vi "Клиент MotorSPS.vi"() -> ()   [LabVIEW 2010]
uses:
  <vilib>/Utility/miscctls.llb/LVScalePositionTypeDef.ctl
  <vilib>/Utility/miscctls.llb/LVRemotePanelConnectionsTypeDef.ctl
panel:
  out "Remote Panel Connections":T1
  out "Remote Panel Controller":i32
  out "VariableIn":T3
  in  "machine name (\"\":  open local reference)":string
  in  "MotorSPS":T4={"Ручной режим управления"={"РучнойСтартСтоп"=FALSE, "Напраление вращения"=enum."Лево", "Время в мин"=18.0, "Поворт экрана"=180.0, "СкорРучРежМот"=0.0, "СкорРучРежРед"=0.0, "Значение энкодера"=0.0, "Расчитать скорость"=FALSE, "Способ управления СПШ"=enum."Управления позицией", "Контроль энкодера"=FALSE, "Инкремент импульсов"=0.0, "Условие энкодер"=FALSE, "Контроль времени"=FALSE, "Лимит времени"=0.0, "Условие время"=FALSE, "Контроль концевиков"=TRUE, "Начальная позиция"=0.0, "Текущая позиция"=0.0, "Выбег"=0.0, "Заданная позиция"=0.0, "Пуск Руч"=FALSE, "Стоп Руч"=FALSE}, "Поиск нулевого положения"={"ИсхСостСтарСтоп"=FALSE, "КонтрольКон"=enum."КонтрольПравКон", "SpeeSlide"=0.0, "Скорость двигателя"=0.0, "Скорость редуктора"=0.0, "Двигатель в исходное сотояние"=FALSE}, "Прав.Конц"=FALSE, "Лев.Конц"=FALSE, "GaugeAngle"={0.0, 0.0}, "Индикатор Статуса Конт"=FALSE, "Статус контроллера СПШ"=enum."Исправен", "Журнал событий"=0, "Выход из программы"=FALSE, "timestamp"=timestamp(0 s since 1904-01-01)} {"timestamp" format="%<%H:%M:%S%3u     %d.%m.%Y>T"; "Поиск нулевого положения"."Скорость двигателя" min=0.0 max=200.0 step=5.0; "Поиск нулевого положения"."SpeeSlide" step=5.0 scale=0.0..200.0; "Ручной режим управления"."Лимит времени" format="%<%M:%S>T"; "Ручной режим управления"."СкорРучРежРед" format="%#_g об/мин"; "Ручной режим управления"."Поворт экрана" min=0.0 max=360.0 step=1.0 format="%#_g °"; "Ручной режим управления"."Время в мин" min=1.0 max=60.0 step=1.0 format="%2d мин"; "Ручной режим управления"."СкорРучРежМот" format="%#_g об/мин"}
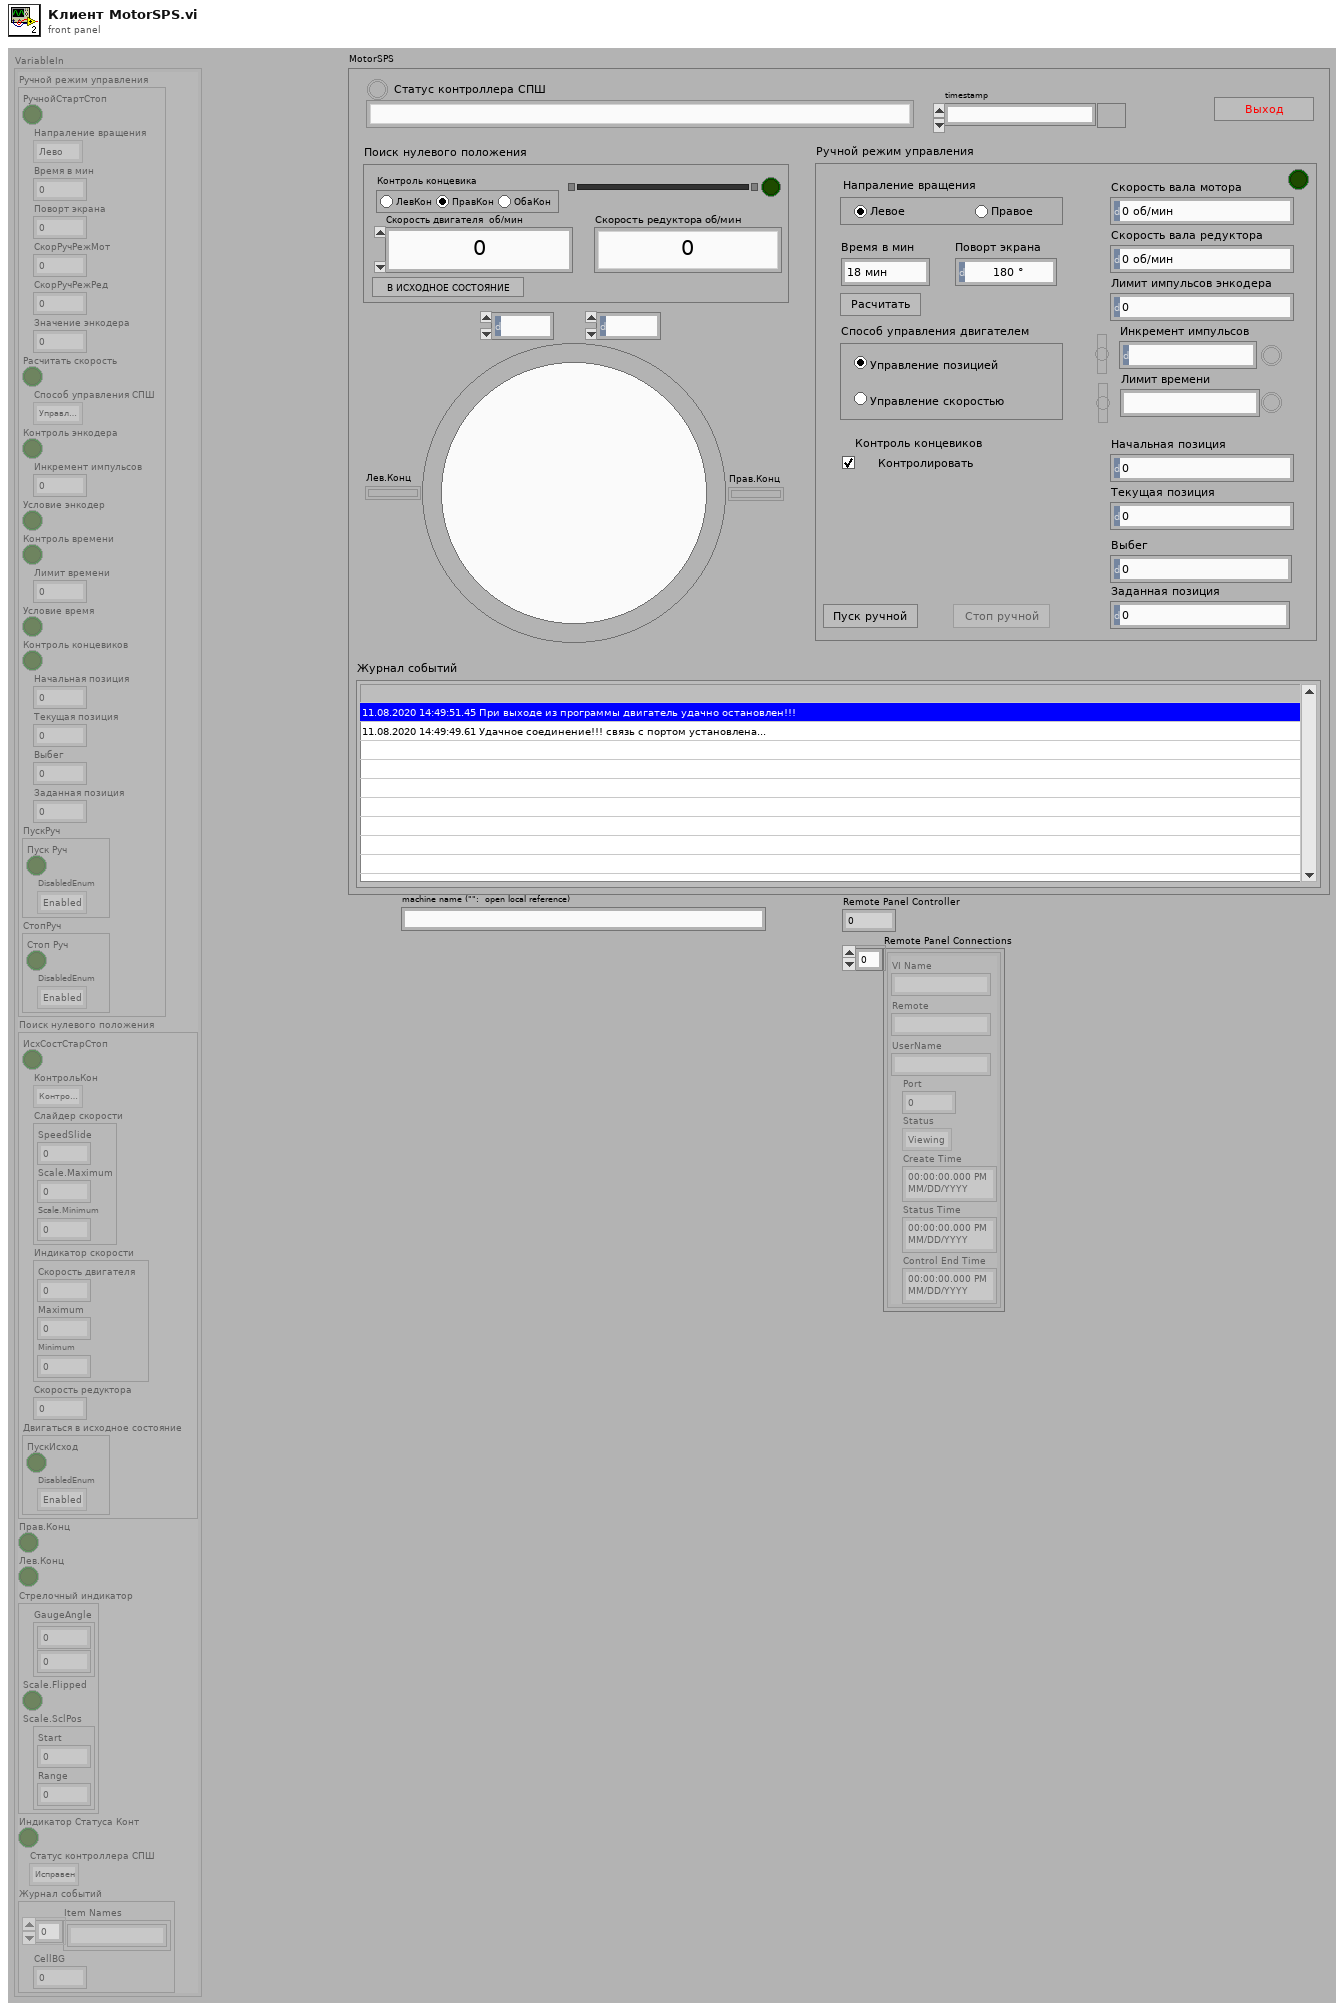
[diagram p1: front panel]
types:
  T1 = typedef "LVRemotePanelConnectionsTypeDef.ctl" = cluster{"VI Name":string, "Remote":string, "UserName":string, "Port":i32, "Status":enum32{"Viewing", "Waiting For Control", "Controlling"}, "Create Time":timestamp, "Status Time":timestamp, "Control End Time":timestamp}[]
  T2 = typedef "LVScalePositionTypeDef.ctl" = cluster{"Start":dbl, "Range":dbl}
  T3 = cluster{"Ручной режим управления":cluster{"РучнойСтартСтоп":bool, "Напраление вращения":enum32{"Лево", "Право"}, "Время в мин":dbl, "Поворт экрана":dbl, "СкорРучРежМот":dbl, "СкорРучРежРед":dbl, "Значение энкодера":dbl, "Расчитать скорость":bool, "Способ управления СПШ":enum32{"Управления позицией", "Управления скоростью"}, "Контроль энкодера":bool, "Инкремент импульсов":dbl, "Условие энкодер":bool, "Контроль времени":bool, "Лимит времени":dbl, "Условие время":bool, "Контроль концевиков":bool, "Начальная позиция":dbl, "Текущая позиция":dbl, "Выбег":dbl, "Заданная позиция":dbl, "ПускРуч":cluster{"Пуск Руч":bool, "DisabledEnum":enum8{"Enabled", "Disabled", "Disabled and Grayed Out"}}, "СтопРуч":cluster{"Стоп Руч":bool, "DisabledEnum":enum8{"Enabled", "Disabled", "Disabled and Grayed Out"}}}, "Поиск нулевого положения":cluster{"ИсхСостСтарСтоп":bool, "КонтрольКон":enum32{"КонтрольЛевКон", "КонтрольПравКон", "КонтрольОбаКон"}, "Слайдер скорости":cluster{"SpeedSlide":dbl, "Scale.Maximum":dbl, "Scale.Minimum":dbl}, "Индикатор скорости":cluster{"Скорость двигателя":dbl, "Maximum":dbl, "Minimum":dbl}, "Скорость редуктора":dbl, "Двигаться в исходное состояние":cluster{"ПускИсход":bool, "DisabledEnum":enum8{"Enabled", "Disabled", "Disabled and Grayed Out"}}}, "Прав.Конц":bool, "Лев.Конц":bool, "Стрелочный индикатор":cluster{"GaugeAngle":cluster{dbl, dbl}, "Scale.Flipped":bool, "Scale.SclPos":T2}, "Индикатор Статуса Конт":bool, "Статус контроллера СПШ":enum16{"Исправен", "Останов по команде", "Останов - высокое противодействующее усилие", "Останов - короткое замыкангие", "Выход из температурного диапазона", "Повышенное силовое напряжение", "Низкое силовое напряжение", "Повышанное цифровое напряжение", "Низкое цифровое напряжение", "Силовое напряжение превышает напряжение, установленое пользователем", "Останов - превышение допустимой перегрузки", "Останов - сработала защита IGBT модуля", "Останов - ощибка поиска фаз по UVW трекам", "Останов - ошибка в настройках энкодера", "Останов - сбой в работе энкодера", "Останов - ошибка фазировки двигателя"}, "Журнал событий":cluster{"Item Names":string[], "CellBG":u32}}
  T4 = cluster{"Ручной режим управления":cluster{"РучнойСтартСтоп":bool, "Напраление вращения":enum32{"Лево", "Право"}, "Время в мин":dbl, "Поворт экрана":dbl, "СкорРучРежМот":dbl, "СкорРучРежРед":dbl, "Значение энкодера":dbl, "Расчитать скорость":bool, "Способ управления СПШ":enum32{"Управления позицией", "Управления скоростью"}, "Контроль энкодера":bool, "Инкремент импульсов":dbl, "Условие энкодер":bool, "Контроль времени":bool, "Лимит времени":dbl, "Условие время":bool, "Контроль концевиков":bool, "Начальная позиция":dbl, "Текущая позиция":dbl, "Выбег":dbl, "Заданная позиция":dbl, "Пуск Руч":bool, "Стоп Руч":bool}, "Поиск нулевого положения":cluster{"ИсхСостСтарСтоп":bool, "КонтрольКон":enum32{"КонтрольЛевКон", "КонтрольПравКон", "КонтрольОбаКон"}, "SpeeSlide":dbl, "Скорость двигателя":dbl, "Скорость редуктора":dbl, "Двигатель в исходное сотояние":bool}, "Прав.Конц":bool, "Лев.Конц":bool, "GaugeAngle":cluster{dbl, dbl}, "Индикатор Статуса Конт":bool, "Статус контроллера СПШ":enum16{"Исправен", "Останов по команде", "Останов - высокое противодействующее усилие", "Останов - короткое замыкангие", "Выход из температурного диапазона", "Повышенное силовое напряжение", "Низкое силовое напряжение", "Повышанное цифровое напряжение", "Низкое цифровое напряжение", "Силовое напряжение превышает напряжение, установленое пользователем", "Останов - превышение допустимой перегрузки", "Останов - сработала защита IGBT модуля", "Останов - ощибка поиска фаз по UVW трекам", "Останов - ошибка в настройках энкодера", "Останов - сбой в работе энкодера", "Останов - ошибка фазировки двигателя"}, "Журнал событий":i32, "Выход из программы":bool, "timestamp":timestamp}
  T5 = cluster{"ИсхСостСтарСтоп":bool, "КонтрольКон":enum32{"КонтрольЛевКон", "КонтрольПравКон", "КонтрольОбаКон"}, "Слайдер скорости":cluster{"SpeedSlide":dbl, "Scale.Maximum":dbl, "Scale.Minimum":dbl}, "Индикатор скорости":cluster{"Скорость двигателя":dbl, "Maximum":dbl, "Minimum":dbl}, "Скорость редуктора":dbl, "Двигаться в исходное состояние":cluster{"ПускИсход":bool, "DisabledEnum":enum8{"Enabled", "Disabled", "Disabled and Grayed Out"}}}
  T6 = cluster{"GaugeAngle":cluster{dbl, dbl}, "Scale.Flipped":bool, "Scale.SclPos":T2}
  T7 = cluster{"РучнойСтартСтоп":bool, "Напраление вращения":enum32{"Лево", "Право"}, "Время в мин":dbl, "Поворт экрана":dbl, "СкорРучРежМот":dbl, "СкорРучРежРед":dbl, "Значение энкодера":dbl, "Расчитать скорость":bool, "Способ управления СПШ":enum32{"Управления позицией", "Управления скоростью"}, "Контроль энкодера":bool, "Инкремент импульсов":dbl, "Условие энкодер":bool, "Контроль времени":bool, "Лимит времени":dbl, "Условие время":bool, "Контроль концевиков":bool, "Начальная позиция":dbl, "Текущая позиция":dbl, "Выбег":dbl, "Заданная позиция":dbl, "ПускРуч":cluster{"Пуск Руч":bool, "DisabledEnum":enum8{"Enabled", "Disabled", "Disabled and Grayed Out"}}, "СтопРуч":cluster{"Стоп Руч":bool, "DisabledEnum":enum8{"Enabled", "Disabled", "Disabled and Grayed Out"}}}
  T8 = enum16{"Исправен", "Останов по команде", "Останов - высокое противодействующее усилие", "Останов - короткое замыкангие", "Выход из температурного диапазона", "Повышенное силовое напряжение", "Низкое силовое напряжение", "Повышанное цифровое напряжение", "Низкое цифровое напряжение", "Силовое напряжение превышает напряжение, установленое пользователем", "Останов - превышение допустимой перегрузки", "Останов - сработала защита IGBT модуля", "Останов - ощибка поиска фаз по UVW трекам", "Останов - ошибка в настройках энкодера", "Останов - сбой в работе энкодера", "Останов - ошибка фазировки двигателя"}
  T9 = enum32{"КонтрольЛевКон", "КонтрольПравКон", "КонтрольОбаКон"}
  T10 = enum8{"Enabled", "Disabled", "Disabled and Grayed Out"}
  T11 = enum32{"Управления позицией", "Управления скоростью"}
  T12 = cluster{"ИсхСостСтарСтоп":bool, "КонтрольКон":enum32{"КонтрольЛевКон", "КонтрольПравКон", "КонтрольОбаКон"}, "SpeeSlide":dbl, "Скорость двигателя":dbl, "Скорость редуктора":dbl, "Двигатель в исходное сотояние":bool}
  T13 = cluster{"РучнойСтартСтоп":bool, "Напраление вращения":enum32{"Лево", "Право"}, "Время в мин":dbl, "Поворт экрана":dbl, "СкорРучРежМот":dbl, "СкорРучРежРед":dbl, "Значение энкодера":dbl, "Расчитать скорость":bool, "Способ управления СПШ":enum32{"Управления позицией", "Управления скоростью"}, "Контроль энкодера":bool, "Инкремент импульсов":dbl, "Условие энкодер":bool, "Контроль времени":bool, "Лимит времени":dbl, "Условие время":bool, "Контроль концевиков":bool, "Начальная позиция":dbl, "Текущая позиция":dbl, "Выбег":dbl, "Заданная позиция":dbl, "Пуск Руч":bool, "Стоп Руч":bool}
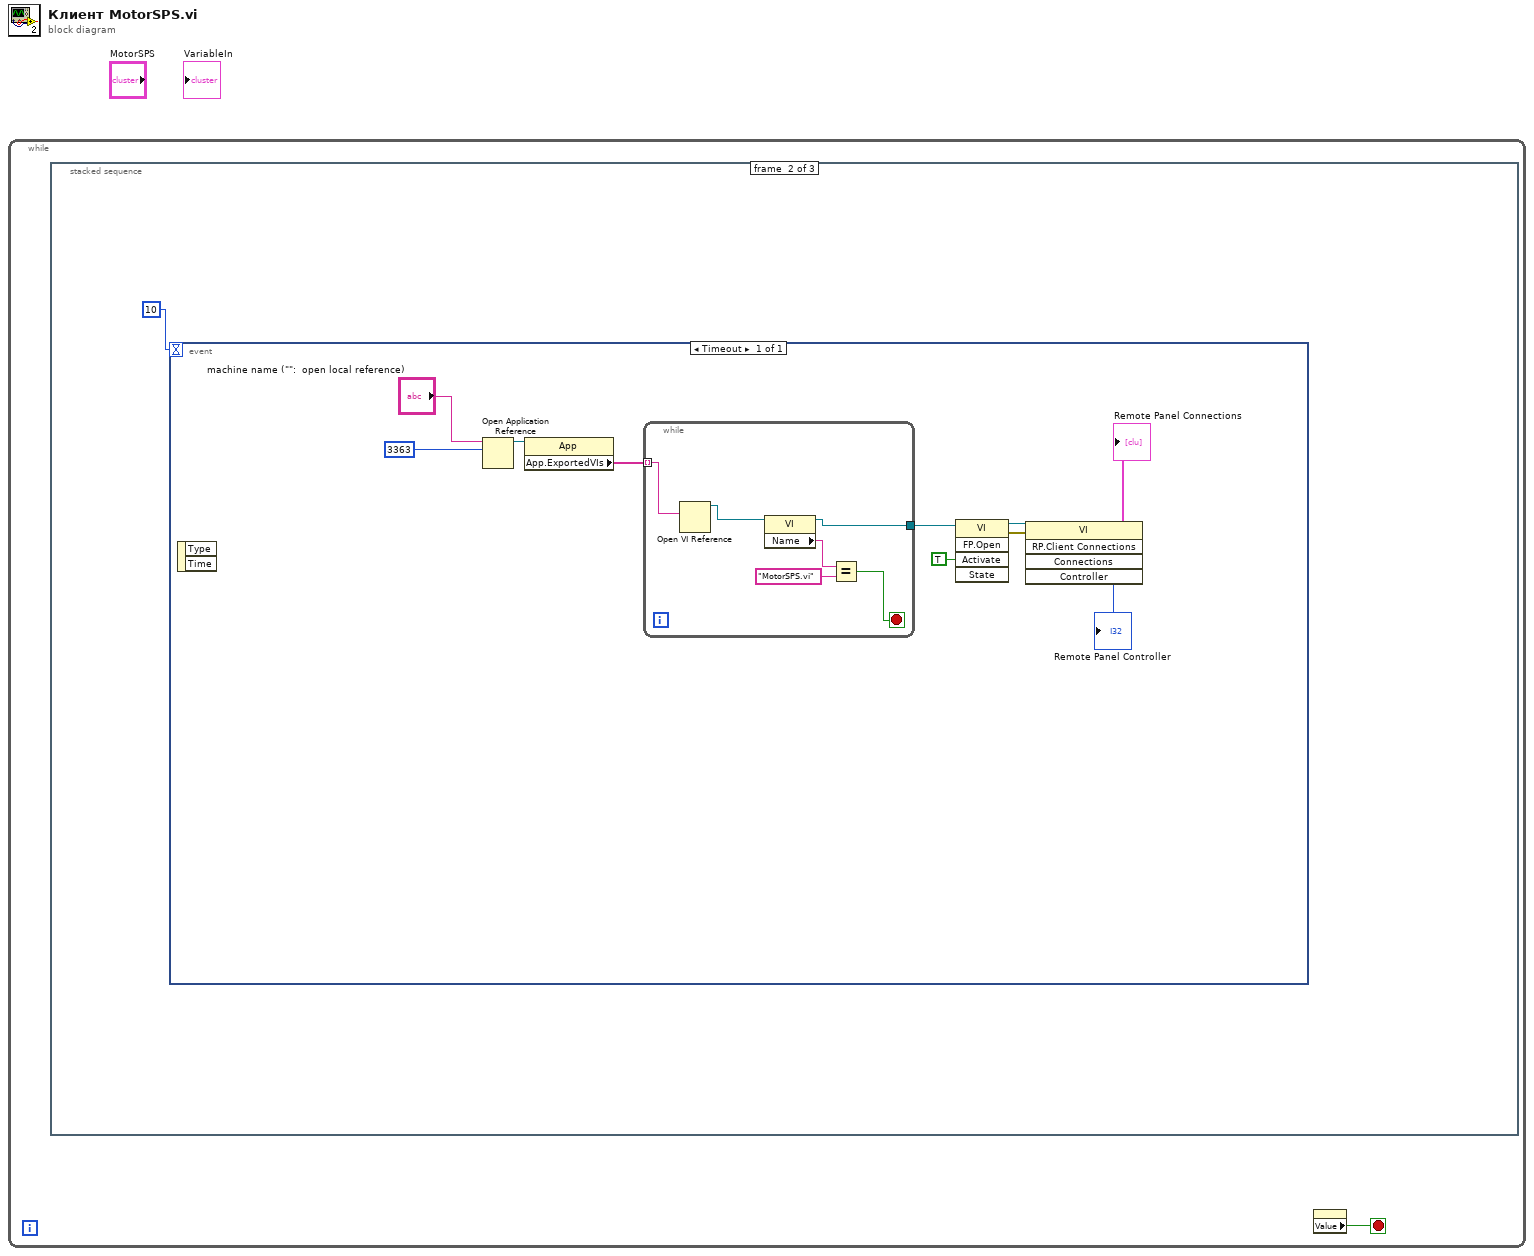
[diagram p0: block diagram]
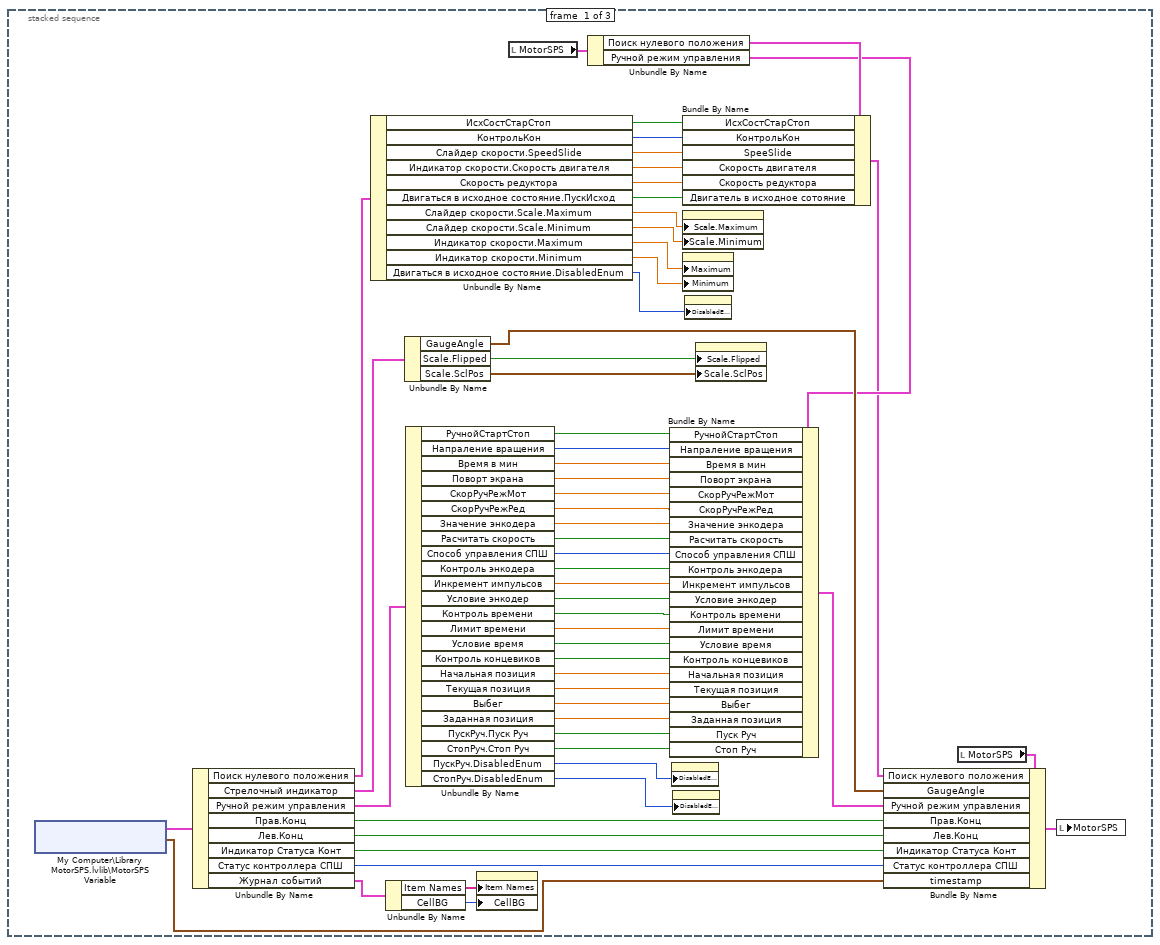
[diagram p2: hidden frame]
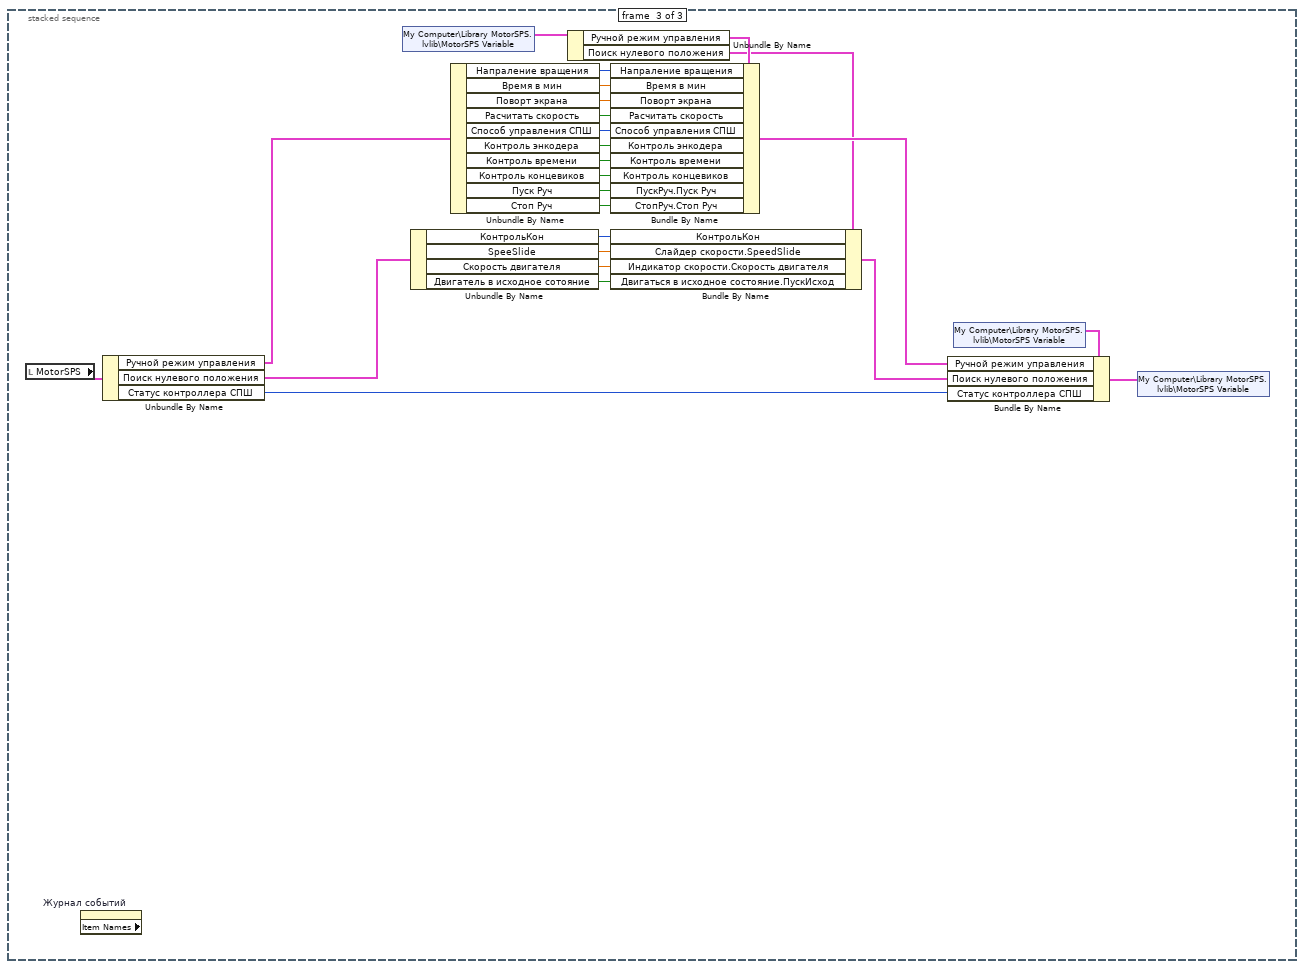
[diagram p3: hidden frame]
diagram:
  n1 = while {
    stop <- w1 stop-if-true
    n2 = stacked-sequence {
      frame #0 {
        n3 = shared-variable "My Computer\\Library MotorSPS.lvlib\\MotorSPS Variable"() -> (w8:T3, w7:timestamp)  [unwired: 1 in, 1 out]
        n4 = Unbundle By Name(w8) -> ("Поиск нулевого положения"=w41:T5, "Стрелочный индикатор"=w40:T6, "Ручной режим управления"=w33:T7, "Прав.Конц"=w37:bool, "Лев.Конц"=w36:bool, "Индикатор Статуса Конт"=w56:bool, "Статус контроллера СПШ"=w55:T8, "Журнал событий"=w54:cluster{"Item Names":string[], "CellBG":u32})
        n5 = Unbundle By Name(w41) -> ("ИсхСостСтарСтоп"=w51:bool, "КонтрольКон"=w50:T9, "Слайдер скорости.SpeedSlide"=w49:dbl, "Индикатор скорости.Скорость двигателя"=w48:dbl, "Скорость редуктора"=w47:dbl, "Двигаться в исходное состояние.ПускИсход"=w46:bool, "Слайдер скорости.Scale.Maximum"=w45:dbl, "Слайдер скорости.Scale.Minimum"=w44:dbl, "Индикатор скорости.Maximum"=w43:dbl, "Индикатор скорости.Minimum"=w42:dbl, "Двигаться в исходное состояние.DisabledEnum"=w35:T10)
        n6 = Unbundle By Name(w54) -> ("Item Names"=w53:string[], "CellBG"=w52:u32)
        n7 = Unbundle By Name(w40) -> ("GaugeAngle"=w39:cluster{dbl, dbl}, "Scale.Flipped"=w38:bool, "Scale.SclPos"=w34:T2)
        n8 = Unbundle By Name(w33) -> ("РучнойСтартСтоп"=w32:bool, "Напраление вращения"=w31:enum32{"Лево", "Право"}, "Время в мин"=w30:dbl, "Поворт экрана"=w29:dbl, "СкорРучРежМот"=w28:dbl, "СкорРучРежРед"=w27:dbl, "Значение энкодера"=w26:dbl, "Расчитать скорость"=w25:bool, "Способ управления СПШ"=w24:T11, "Контроль энкодера"=w23:bool, "Инкремент импульсов"=w22:dbl, "Условие энкодер"=w21:bool, "Контроль времени"=w20:bool, "Лимит времени"=w19:dbl, "Условие время"=w18:bool, "Контроль концевиков"=w17:bool, "Начальная позиция"=w16:dbl, "Текущая позиция"=w15:dbl, "Выбег"=w14:dbl, "Заданная позиция"=w13:dbl, "ПускРуч.Пуск Руч"=w12:bool, "СтопРуч.Стоп Руч"=w11:bool, "ПускРуч.DisabledEnum"=w10:T10, "СтопРуч.DisabledEnum"=w9:T10)
        n9 = property on="Журнал событий" class="LstBox (strict)"("Item Names"=w53, "CellBG"=w52) -> ()  [unwired: 2 in, 2 out]
        n10 = local read "MotorSPS"() -> (w6:T4)
        n11 = Unbundle By Name(w6) -> ("Поиск нулевого положения"=w5:T12, "Ручной режим управления"=w4:T13)
        n12 = Bundle By Name(cluster=w4, "РучнойСтартСтоп"=w32, "Напраление вращения"=w31, "Время в мин"=w30, "Поворт экрана"=w29, "СкорРучРежМот"=w28, "СкорРучРежРед"=w27, "Значение энкодера"=w26, "Расчитать скорость"=w25, "Способ управления СПШ"=w24, "Контроль энкодера"=w23, "Инкремент импульсов"=w22, "Условие энкодер"=w21, "Контроль времени"=w20, "Лимит времени"=w19, "Условие время"=w18, "Контроль концевиков"=w17, "Начальная позиция"=w16, "Текущая позиция"=w15, "Выбег"=w14, "Заданная позиция"=w13, "Пуск Руч"=w12, "Стоп Руч"=w11) -> (w3:T13)
        n13 = property on="Пуск Руч" class="Bool (strict)"("DisabledEnum"=w10) -> ()  [unwired: 2 in, 2 out]
        n14 = property on="Стоп Руч" class="Bool (strict)"("DisabledEnum"=w9) -> ()  [unwired: 2 in, 2 out]
        n15 = Bundle By Name(cluster=w5, "ИсхСостСтарСтоп"=w51, "КонтрольКон"=w50, "SpeeSlide"=w49, "Скорость двигателя"=w48, "Скорость редуктора"=w47, "Двигатель в исходное сотояние"=w46) -> (w2:T12)
        n16 = property on="SpeeSlide" class="Slide (strict)"("Scale.Maximum"=w45, "Scale.Minimum"=w44) -> ()  [unwired: 2 in, 2 out]
        n17 = property on="Скорость двигателя" class="DigNum (strict)"("Maximum"=w43, "Minimum"=w42) -> ()  [unwired: 2 in, 2 out]
        n18 = property on="Двигатель в исходное сотояние" class="Bool (strict)"("DisabledEnum"=w35) -> ()  [unwired: 2 in, 2 out]
        n19 = property on="GaugeAngle" class="Knob (strict)"("Scale.Flipped"=w38, "Scale.SclPos"=w34) -> ()  [unwired: 2 in, 2 out]
        n20 = local read "MotorSPS"() -> (w57:T4)
        n21 = Bundle By Name(cluster=w57, "Поиск нулевого положения"=w2, "GaugeAngle"=w39, "Ручной режим управления"=w3, "Прав.Конц"=w37, "Лев.Конц"=w36, "Индикатор Статуса Конт"=w56, "Статус контроллера СПШ"=w55, "timestamp"=w7) -> (w58:T4)
        n22 = local write "MotorSPS"(w58) -> ()
      }
      frame #1 {
        n23 = event shown="[0] Timeout" {
          selector: _ -> [_]
          dyn-events: _ -> [_]
          timeout: 10 -> [_]
          event Timeout {
            n24 = event-data() -> ()  [unwired: 1 in, 2 out]
            n25 = Open Application Reference(10:u16 3363 ("port number or service name (3363)"), 11:"machine name (\"\":  open local reference)") -> (3:w67:refnum<vi>)  [unwired: 2 in, 1 out]
            n26 = property class="App"(reference=w67) -> ("App.ExportedVIs"=w66:string[])  [unwired: 1 in, 2 out]
            n27 = while {
              tunnel: w66 -> [w75] mode=indexing
              tunnel: [w70] -> w65
              stop <- w71 stop-if-true
              n28 = Open VI Reference(vi path=w75) -> (vi reference=w74:refnum<vi>)  [unwired: 5 in, 1 out]
              n29 = property class="VI"(reference=w74) -> (reference out=w70:refnum<vi>, "Name"=w73:string)  [unwired: 1 in, 1 out]
              n30 = Equal?(x=w73, y="MotorSPS.vi") -> (x = y?=w71:bool)
            }
            n31 = invoke class="VI" method="FP.Open"(reference=w65, "Activate"=TRUE ("Activate?")) -> (reference out=w63:refnum<vi>, error out=w62:errorcluster)  [unwired: 3 in, 3 out]
            n32 = invoke class="VI" method="RP.Client Connections"(reference=w63, error in=w62) -> ("Connections"=→"Remote Panel Connections":T1, "Controller"=→"Remote Panel Controller":i32)  [unwired: 3 in, 3 out]
          }
        }
      }
      frame #2 {
        n33 = local read "MotorSPS"() -> (w100:T4)
        n34 = property on="Журнал событий" class="LstBox (strict)" props=["Item Names"]() -> ()  [unwired: 2 in, 3 out]
        n35 = Unbundle By Name(w100) -> ("Ручной режим управления"=w99:T13, "Поиск нулевого положения"=w88:T12, "Статус контроллера СПШ"=w82:T8)
        n36 = shared-variable "My Computer\\Library MotorSPS.lvlib\\MotorSPS Variable"() -> (w80:T3)  [unwired: 1 in, 1 out]
        n37 = Unbundle By Name(w88) -> ("КонтрольКон"=w87:T9, "SpeeSlide"=w86:dbl, "Скорость двигателя"=w85:dbl, "Двигатель в исходное сотояние"=w84:bool)
        n38 = Unbundle By Name(w99) -> ("Напраление вращения"=w98:enum32{"Лево", "Право"}, "Время в мин"=w97:dbl, "Поворт экрана"=w96:dbl, "Расчитать скорость"=w95:bool, "Способ управления СПШ"=w94:T11, "Контроль энкодера"=w93:bool, "Контроль времени"=w92:bool, "Контроль концевиков"=w91:bool, "Пуск Руч"=w90:bool, "Стоп Руч"=w89:bool)
        n39 = Unbundle By Name(w80) -> ("Ручной режим управления"=w78:T7, "Поиск нулевого положения"=w77:T5)
        n40 = Bundle By Name(cluster=w78, "Напраление вращения"=w98, "Время в мин"=w97, "Поворт экрана"=w96, "Расчитать скорость"=w95, "Способ управления СПШ"=w94, "Контроль энкодера"=w93, "Контроль времени"=w92, "Контроль концевиков"=w91, "ПускРуч.Пуск Руч"=w90, "СтопРуч.Стоп Руч"=w89) -> (w79:T7)
        n41 = Bundle By Name(cluster=w77, "КонтрольКон"=w87, "Слайдер скорости.SpeedSlide"=w86, "Индикатор скорости.Скорость двигателя"=w85, "Двигаться в исходное состояние.ПускИсход"=w84) -> (w83:T5)
        n42 = shared-variable "My Computer\\Library MotorSPS.lvlib\\MotorSPS Variable"() -> (w81:T3)  [unwired: 1 in, 1 out]
        n43 = Bundle By Name(cluster=w81, "Ручной режим управления"=w79, "Поиск нулевого положения"=w83, "Статус контроллера СПШ"=w82) -> (w76:T3)
        n44 = shared-variable "My Computer\\Library MotorSPS.lvlib\\MotorSPS Variable"(w76) -> ()  [unwired: 1 in, 1 out]
      }
    }
    n45 = property on="Выход из программы" class="Bool (strict)"() -> ("Value"=w1:bool)  [unwired: 2 in, 2 out]
  }
